vi "Turret_Execute.vi"() -> ()   [LabVIEW 2020]
uses:
  Turret_States.ctl
  Globals/Turret_Globals.vi
  Globals/Sensor_Values.vi
  <vilib>/Rock Robotics/WPI/ThirdParty/Phoenix-LabVIEW/Motor Controller/Controls/CTRE_Phoenix_MotorControl_ControlMode.ctl
panel:
  in  "Disable Edge Safeties?":bool
  out "Waveform Chart":cluster{"Goal Wheel Position":dbl, dbl}(graph)
  in  "Kp_Degrees":dbl=0.07
  in  "Kd Aim":dbl=0.001
  in  "Ki Aim":dbl=1e-05
  in  "upper_limit(degrees)":dbl=160.0
  in  "lower_limit(degrees)":dbl=-160.0
  out "Turret_Spin_Speed":dbl
  in  "Kp Aim":dbl=0.06
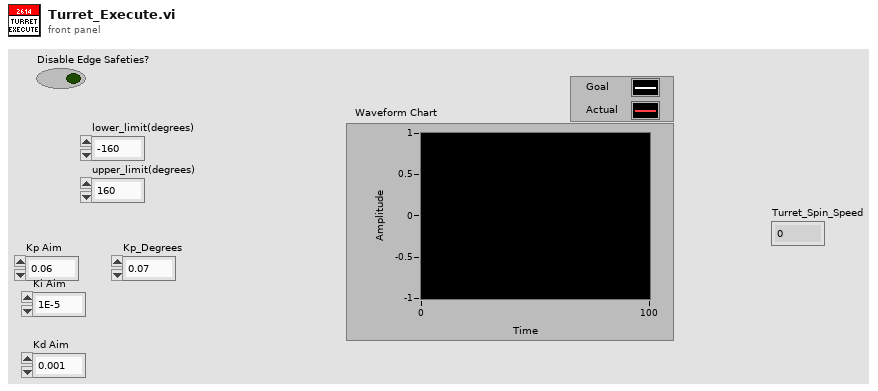
[diagram p1: front panel]
types:
  T1 = typedef "Turret_States.ctl" = enum16{"Manual_Percent_Voltage", "Manual_Speed_Control", "Auto-Target", "Command_TurnToPosition", "Command_Auto_Target", "GoToZero", "No-Op"}
  T2 = typedef "Turret_Cluster.ctl" = cluster{"Turret_Control_State":T1, "Manual_Speed":dbl, "Step":i32, "Parameter_1":dbl, "Parameter_2":dbl, "Parameter_3":dbl, "Auto_Notifier":refnum<notifier>, "Goal_Angle":dbl, "Camera_Goal_X":dbl}
  T3 = typedef "CTRE_Phoenix_MotorControl_ControlMode.ctl" = u16
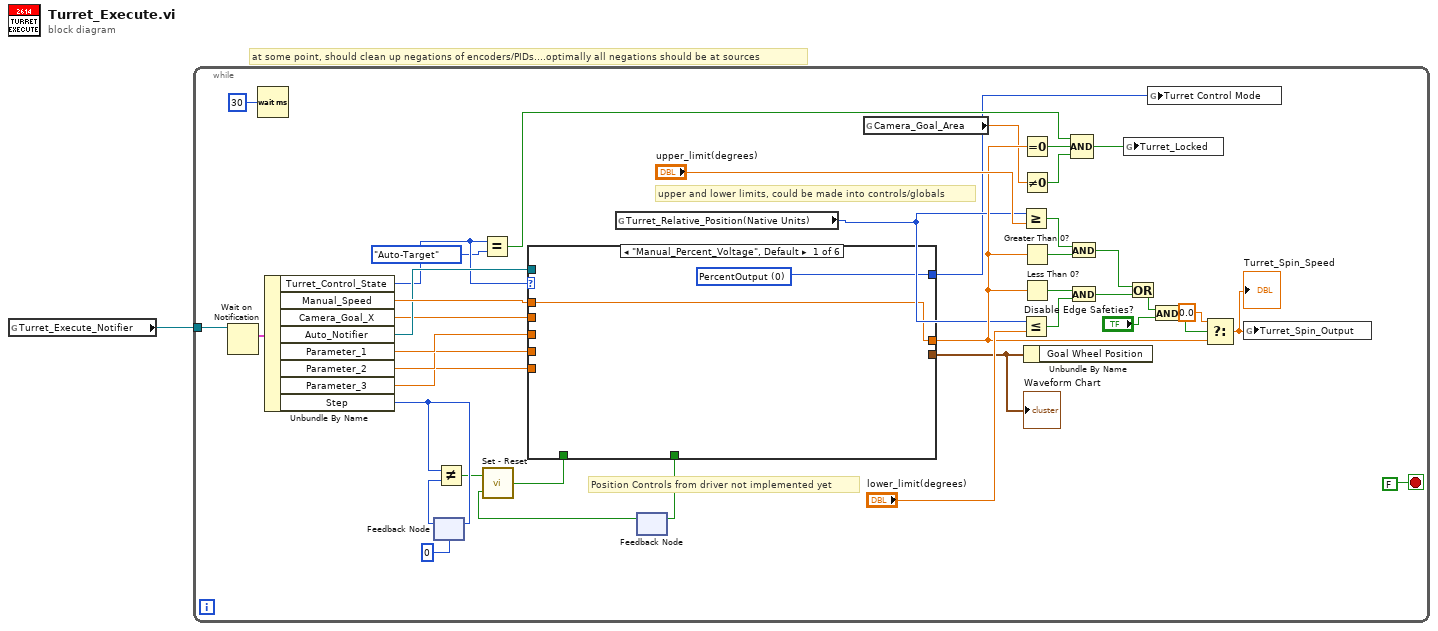
[diagram p0: block diagram]
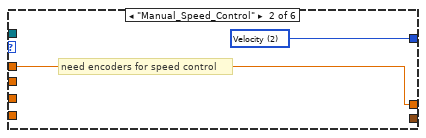
[diagram p2: hidden frame]
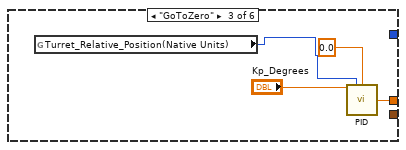
[diagram p3: hidden frame]
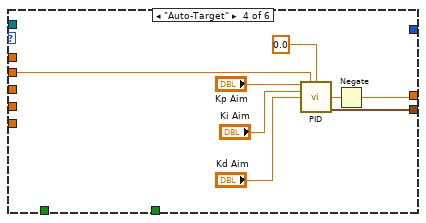
[diagram p4: hidden frame]
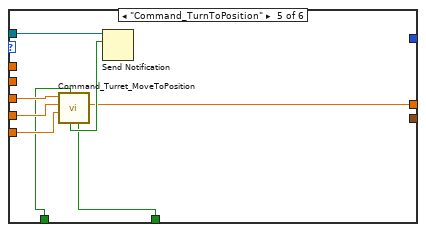
[diagram p5: hidden frame]
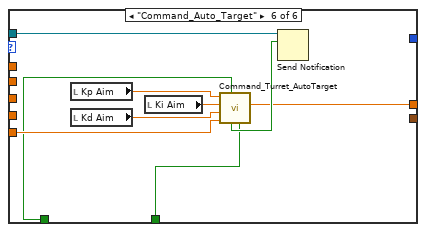
[diagram p6: hidden frame]
diagram:
  # "at some point, should clean up negations of encoders/PIDs....optimally all negations should be at sources"
  n1 = global read "Turret_Globals.vi" "Turret_Execute_Notifier"() -> (w1:refnum<notifier>)
  n2 = while {
    tunnel: w1 -> [w41]
    stop <- FALSE stop-if-true
    # "Position Controls from driver not implemented yet"
    # "upper and lower limits, could be made into controls/globals"
    n3 = Wait on Notification(notifier=w41) -> (notification=w40:T2)  [unwired: 3 in, 3 out]
    n4 = Wait (ms)(milliseconds to wait=u32 30) -> ()  [unwired: 1 out]
    n5 = Unbundle By Name(w40) -> ("Turret_Control_State"=w23:T1, "Manual_Speed"=w39:dbl, "Camera_Goal_X"=w2:dbl, "Auto_Notifier"=w24:refnum<notifier>, "Parameter_1"=w28:dbl, "Parameter_2"=w27:dbl, "Parameter_3"=w26:dbl, "Step"=w6:i32)
    n6 = feedback #1(0 ("Step")) -> (w8:i32)
    n7 = feedback-in #1(w6) -> ()
    n8 = Not Equal?(x=w6, y=w8) -> (x != y?=w5:bool)
    n9 = Equal?(x=w23, y=Turret_States."Auto-Target") -> (x = y?=w19:bool)
    n10 = global read "Sensor_Values.vi" "Turret_Relative_Position(Native Units)"() -> (w10:i32)
    n11 = feedback #2() -> (w3:bool)  [unwired: 1 in]
    n12 = call "Set - Reset.vi"("Reset"=w3, "Set"=w5) -> ("Output"=w25:bool)
    n13 = case shown="\"Manual_Percent_Voltage\", Default" w23 {
      tunnel: w39 -> [w44 w46 _ _ _ _]
      tunnel: [w44 w46 w48 w52 w59 w67] -> w21
      tunnel: w28 -> [_ _ _ _ w66 _]
      tunnel: w27 -> [_ _ _ _ w65 _]
      tunnel: w26 -> [_ _ _ _ w64 w72]
      tunnel: w25 -> [_ _ _ _ w63 w71]
      tunnel: w24 -> [_ _ _ _ w62 w70]
      tunnel: [_ _ _ _ w60 w68] -> w4
      tunnel: [_ _ _ w54 _ _] -> w15
      tunnel: [w43 w45 _ _ _ _] -> w9
      tunnel: w2 -> [_ _ _ w51 _ _]
      frame "Manual_Percent_Voltage", Default {
        w43 = T3 0 items=["PercentOutput"=0, "Position"=1, "Velocity"=2, "Current"=3, "Follower"=5, "MotionProfile"=6, "MotionMagic"=7, "MotionProfileArc"=10, "Disabled"=15] ("Control Mode")
      }
      frame "Manual_Speed_Control" {
        w45 = T3 2 items=["PercentOutput"=0, "Position"=1, "Velocity"=2, "Current"=3, "Follower"=5, "MotionProfile"=6, "MotionMagic"=7, "MotionProfileArc"=10, "Disabled"=15] ("Control Mode")
        # "need encoders for speed control"
      }
      frame "GoToZero" {
        n14 = global read "Sensor_Values.vi" "Turret_Relative_Position(Native Units)"() -> (w47:i32)
        n15 = call "PID.vi"("Kp"="Kp_Degrees", "Process Variable"=w47, "Goal"=0.0) -> ("Command"=w48:dbl)  [unwired: 10 in, 2 out]
      }
      frame "Auto-Target" {
        n16 = call "PID.vi"("Kp"="Kp Aim", "Process Variable"=w51, "Goal"=0.0, "Ki"="Ki Aim", "Kd"="Kd Aim") -> ("Command"=w53:dbl, "PID Tracking"=w54:cluster{"Goal Wheel Position":dbl, dbl})  [unwired: 8 in, 1 out]
        n17 = Negate(x=w53) -> (-x=w52:dbl)
      }
      frame "Command_TurnToPosition" {
        n18 = call "Command_Turret_MoveToPosition.vi"("Startup"=w63, "Timeout"=w64, "Speed"=w65, "Goal_Position"=w66) -> ("Turret_Speed"=w59:dbl, "Reint"=w60:bool, "Completed"=w61:bool)  [unwired: 5 in]
        n19 = Send Notification(notification=w61, notifier=w62) -> ()  [unwired: 1 in, 2 out]
      }
      frame "Command_Auto_Target" {
        n20 = local read "Kp Aim"() -> (w75:dbl)
        n21 = local read "Kd Aim"() -> (w73:dbl)
        n22 = local read "Ki Aim"() -> (w74:dbl)
        n23 = call "Command_Turret_AutoTarget.vi"("Startup"=w71, "Timeout"=w72, "Kd"=w73, "Ki"=w74, "Kp"=w75) -> ("Turret_Speed"=w67:dbl, "Reint"=w68:bool, "Completed"=w69:bool)  [unwired: 4 in]
        n24 = Send Notification(notification=w69, notifier=w70) -> ()  [unwired: 1 in, 2 out]
      }
    }
    "Waveform Chart" <- w15
    n25 = feedback-in #2(w4) -> ()
    n26 = global read "Sensor_Values.vi" "Camera_Goal_Area"() -> (w17:dbl)
    n27 = Greater Or Equal?(x=w10, y="upper_limit(degrees)") -> (x >= y?=w38:bool)
    n28 = Less Or Equal?(x=w10, y="lower_limit(degrees)") -> (x <= y?=w31:bool)
    n29 = Equal To 0?(x=w21) -> (x = 0?=w18:bool)
    n30 = Not Equal To 0?(x=w17) -> (x != 0?=w16:bool)
    n31 = Greater Than 0?(x=w21) -> (x > 0?=w37:bool)
    n32 = Less Than 0?(x=w21) -> (x < 0?=w36:bool)
    n33 = Unbundle By Name(w15) -> ()  [unwired: 1 out]
    n34 = And(x=w38, y=w37) -> (x .and. y?=w34:bool)
    n35 = And(x=w36, y=w31) -> (x .and. y?=w35:bool)
    n36 = Compound Arithmetic op=AND(w19, w18, w16) -> (w20:bool)
    n37 = global write "Turret_Globals.vi" "Turret_Locked"(w20) -> ()
    n38 = Or(x=w34, y=w35) -> (x .or. y?=w13:bool)
    n39 = global write "Turret_Globals.vi" "Turret Control Mode"(w9) -> ()
    n40 = And(x=w13, y="Disable Edge Safeties?") -> (x .and. y?=w11:bool)
    n41 = Select(t=0.0, s=w11, f=w21) -> (s? t:f=w14:dbl)
    "Turret_Spin_Speed" <- w14
    n42 = global write "Turret_Globals.vi" "Turret_Spin_Output"(w14) -> ()
  }
